vi "cc_init.vi"(7 "Serial Configuration":cluster{"Baud Rate":u32}={"Baud Rate"=9600} {"Baud Rate" items=["300"=300, "600"=600, "1200"=1200, "2400"=2400, "4800"=4800, "9600"=9600, "19200"=19200]}, 8 "error in (no error)":errorcluster, 11 "VISA resource name":refnum<visa-resource-name>="tcpip0::192.168.1.5::5000::SOCKET") -> (0 "error out":errorcluster, 3 "VISA resource name out":refnum<visa-resource-name>)   [LabVIEW 2020]
doc: "Establishes communication with the instrument and optionally performs an instrument identification query and/or an instrument reset. It also places the instrument in a default state needed for other instrument driver operations. Therefore, call this VI before calling other instrument driver VIs for this instrument. Generally, you need to call the Initialize VI only once at the beginning of an application."
panel:
  out "IDN String":string
  # "(c) 2011. Cryogenic Control Systems, Inc..  ALL RIGHTS RESERVED."
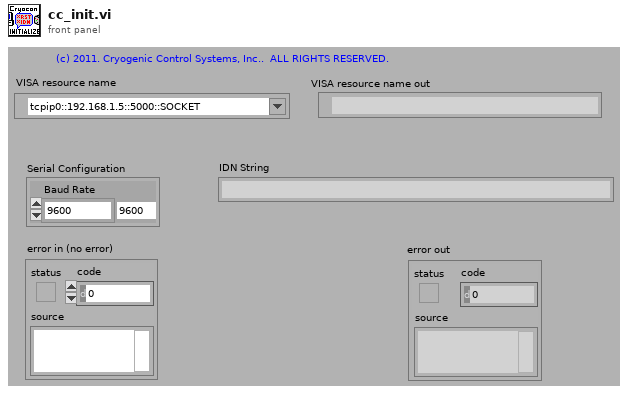
[diagram p1: front panel]
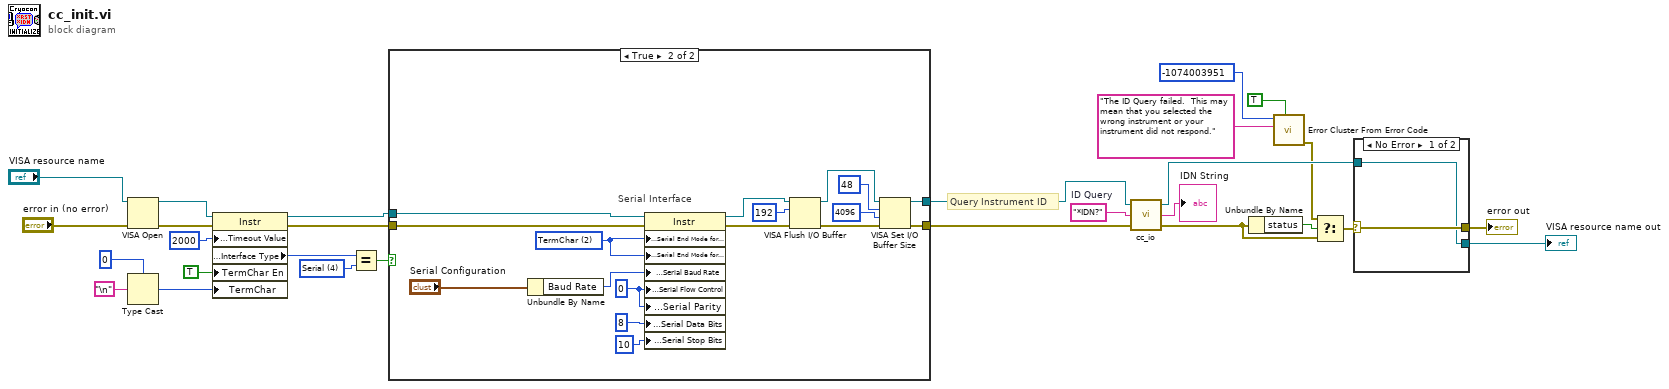
[diagram p0: block diagram]
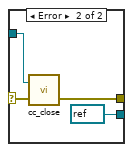
[diagram p3: hidden frame]
diagram:
  w9 = "*IDN?"  # ID Query
  w19 = u16 4 items=["GPIB"=1, "VXI"=2, "GPIB-VXI"=3, "Serial"=4, "PXI"=5, "TCPIP"=6, "USB"=7] ("Interface Information:Interface Type")
  # "Query Instrument ID"
  n1 = VISA Open(error in (no error)="error in (no error)", VISA resource name="VISA resource name") -> (VISA resource name=w14:refnum<visa-resource-name>, error out=w13:errorcluster)  [unwired: 3 in]
  n2 = Type Cast(type=u8 0, x="\n" ("Line Feed Constant")) -> (*(type *) &x=w1:u8)
  n3 = property class="Instr"(reference=w14, error in=w13, "General Settings:Timeout Value"=u32 2000, "TermChar En"=TRUE ("Message Based Settings:Termination Character Enable"), "TermChar"=w1) -> (reference out=w22:refnum<visa-resource-name>, error out=w21:errorcluster, "Interface Information:Interface Type"=w26:u16)
  n4 = Equal?(x=w26, y=w19) -> (x = y?=w20:bool)
  n5 = case shown="True" w20 {
    tunnel: [w29 w44] -> w24
    tunnel: [w30 w41] -> w23
    tunnel: w22 -> [w29 w46]
    tunnel: w21 -> [w30 w47]
    frame False {
      # "TCP/IP uses end-of-line char of \\n to terminate reads"
      # "GPIB and TCP/IP Interfaces"
    }
    frame True {
      w33 = u16 0
      w36 = u16 2 items=["None", "LastBit", "TermChar"] ("Serial Settings:Serial End Mode for Reads")
      # "Serial Interface"
      n6 = Unbundle By Name("Serial Configuration") -> ("Baud Rate"=w35:u32)
      n7 = property class="Instr"(reference=w46, error in=w47, "Serial Settings:Serial End Mode for Reads"=w36, "Serial Settings:Serial End Mode for Writes"=w36, "Serial Settings:Serial Baud Rate"=w35, "Serial Settings:Serial Flow Control"=w33, "Serial Settings:Serial Parity"=w33, "Serial Settings:Serial Data Bits"=u16 8, "Serial Settings:Serial Stop Bits"=u16 10) -> (reference out=w40:refnum<visa-resource-name>, error out=w43:errorcluster)
      n8 = VISA Flush I/O Buffer(VISA resource name=w40, mask (16)=u16 192, error in (no error)=w43) -> (VISA resource name out=w45:refnum<visa-resource-name>, error out=w42:errorcluster)
      n9 = VISA Set I/O Buffer Size(VISA resource name=w45, mask (16)=u16 48, size (4096)=u32 4096 ("size (0)"), error in (no error)=w42) -> (VISA resource name out=w44:refnum<visa-resource-name>, error out=w41:errorcluster)
    }
  }
  n10 = call "cc_io.vi"("error in (no error)"=w23, "Output Command"=w9, "VISA In"=w24) -> ("error out"=w4:errorcluster, "Input String"=→"IDN String":string, "VISA out"=w16:refnum<visa-resource-name>)
  n11 = Unbundle By Name(w4) -> ("status"=w8:bool)
  n12 = call <vilib>:"Error Cluster From Error Code.vi"("show call chain? (False)"=TRUE, "error message (\"\")"="The ID Query failed.  This may mean that you selected the wrong instrument or your instrument did not respond." ("Source (VI Name)"), "error code (0)"=-1074003951 ("Code")) -> ("error out"=w5:errorcluster)  [unwired: 6 in]
  n13 = Select(t=w5, s=w8, f=w4) -> (s? t:f=w15:errorcluster)
  n14 = case shown="No Error" w15 {
    selector: w15 -> [w49 w52]
    tunnel: [w48 refnum<visa-resource-name> refnum ("VISA resource name out")] -> w18
    tunnel: [w49 w53] -> w17
    tunnel: w16 -> [w48 w50]
    frame No Error {
    }
    frame Error {
      n15 = call "cc_close.vi"("error in (no error)"=w52, "VISA In"=w50) -> ("error out"=w53:errorcluster)  [unwired: 1 in]
    }
  }
  "VISA resource name out" <- w18
  "error out" <- w17
